vi "BuildPathPointTable.vi"(8 "error in":T1, 10 "yCoordinates":sgl[](array[numeric])=[8.0, 9.0, 10.0, 11.0, 12.0, 13.0, 14.0] format="%#_g µm", 11 "xCoordinates":sgl[](array[numeric])=[1.0, 2.0, 3.0, 4.0, 5.0, 6.0, 7.0] format="%#_g µm") -> (0 "error out":T1, 3 "PathPoints":string[][](table))   [LabVIEW 2016]
uses:
  Controls/Error_Out.ctl
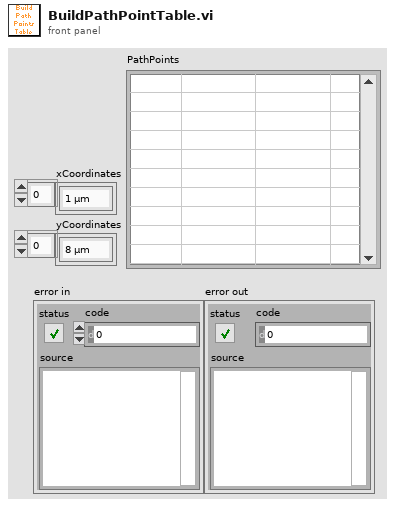
[diagram p1: front panel]
types:
  T1 = typedef "Error_Out.ctl" = errorcluster
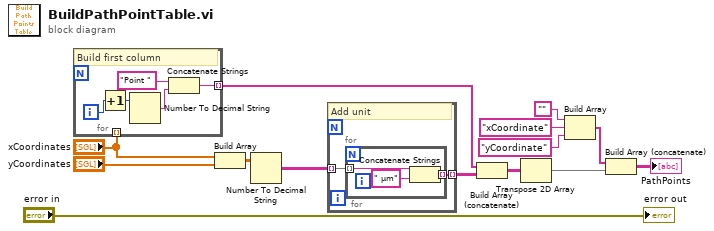
[diagram p0: block diagram]
diagram:
  n1 = for {
    tunnel: "xCoordinates" -> [_] mode=indexing
    tunnel: [w17] -> w11 mode=indexing
    i -> [w16]
    # "Build first column"
    n2 = Increment(x=w16) -> (x+1=w15:i32)
    n3 = Number To Decimal String(number=w15) -> (decimal integer string=w18:string)  [unwired: 1 in]
    n4 = Concatenate Strings("Point ", w18) -> (w17:string)
  }
  n5 = Build Array("xCoordinates", "yCoordinates") -> (w12:sgl[][])
  n6 = Number To Decimal String(number=w12) -> (decimal integer string=w2:string[][])  [unwired: 1 in]
  n7 = for {
    tunnel: w2 -> [w21] mode=indexing
    tunnel: [w20] -> w1 mode=indexing
    # "Add unit"
    n8 = for {
      tunnel: w21 -> [w24] mode=indexing
      tunnel: [w22] -> w20 mode=indexing
      n9 = Concatenate Strings(w24, " µm" ("string")) -> (w22:string)
    }
  }
  n10 = Build Array (concatenate)(w11, w1) -> (w10:string[][])
  n11 = Transpose 2D Array(2D array=w10) -> (transposed array=w6:string[][])
  n12 = Build Array("", "xCoordinate", "yCoordinate") -> (w7:string[])
  n13 = Build Array (concatenate)(w7, w6) -> (→"PathPoints":string[][])
  "error out" <- "error in"
